vi "Acquire.vi"(8 "error in (no error)":errorcluster, 10 "Msg in":T1, 11 "PXIDigitizer in":refnum<class "PXIDigitizer.lvclass">) -> (0 "error out":errorcluster, 1 "new command":string, 2 "Msg out":T1, 3 "PXIDigitizer out":refnum<class "PXIDigitizer.lvclass">)   [LabVIEW 2011, in "PXIDigitizer.lvclass"]
uses:
  PXIDigitizer.lvclass
  DriverMsg.ctl
  PXIDigitizer.lvclass/PXIDigitizer.ctl
  BaseDriver/BaseDriver.lvclass
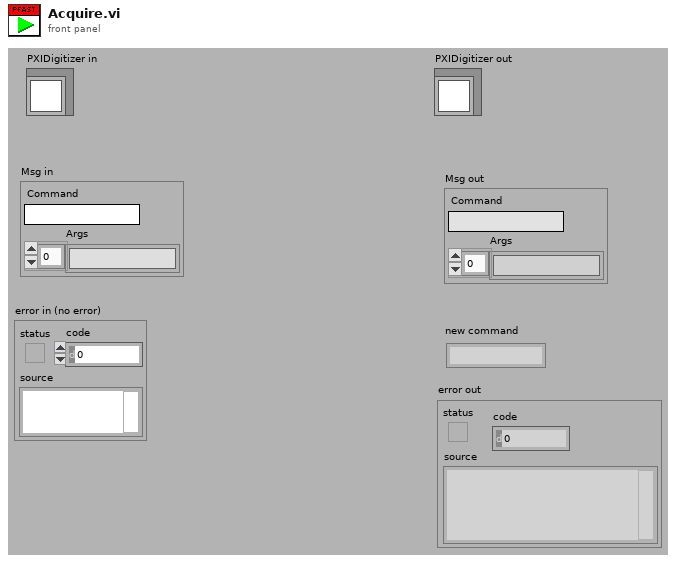
[diagram p1: front panel]
types:
  T1 = typedef "DriverMsg.ctl" = cluster{"Command":string, "Args":string[]}
  T2 = typedef "OnOffTypeDef.ctl" = enum16{"off", "on"}
  T3 = typedef "methodCluster_TypDEf.ctl" = cluster{"Analysis1":T4, "Analysis2":T4, "Analysis3":T4, "Analysis4":T4, "Analysis5":T4, "Analysis6":T4, "Analysis7":T4, "Analysis8":T4, "Analysis9":T4, "Analysis10":T4}
  T4 = typedef "method_TypDef.ctl" = enum16{"n/a", "max", "min", "energy"}
  T5 = typedef "LinkedChannelsCluster_TypDef.ctl" = cluster{"Analysis1":T6, "Analysis2":T6, "Analysis3":T6, "Analysis4":T6, "Analysis5":T6, "Analysis6":T6, "Analysis7":T6, "Analysis8":T6, "Analysis9":T6, "Analysis10":T6}
  T6 = typedef "channels_TypDef.ctl" = enum16{"Channel0", "Channel1", "Channel2", "Channel3", "Channel4", "Channel5", "Channel6", "Channel7", "n/a"}
  T7 = typedef "MeasurementsCluster_TypDEf.ctl" = cluster{"Analysis1":dbl, "Analysis2":dbl, "Analysis3":dbl, "Analysis4":dbl, "Analysis5":dbl, "Analysis6":dbl, "Analysis7":dbl, "Analysis8":dbl, "Analysis9":dbl, "Analysis10":dbl}
  T8 = cluster{"actualSamples":i32, "absoluteInitialX":dbl, "relativeInitialX":dbl, "xIncrement":dbl, "offset":dbl, "gain":dbl, "reserved1":dbl, "reserved2":dbl}[]
  T9 = cluster{"Channel0":string, "Channel1":string, "Channel2":string, "Channel3":string, "Channel4":string, "Channel5":string, "Channel6":string, "Channel7":string}
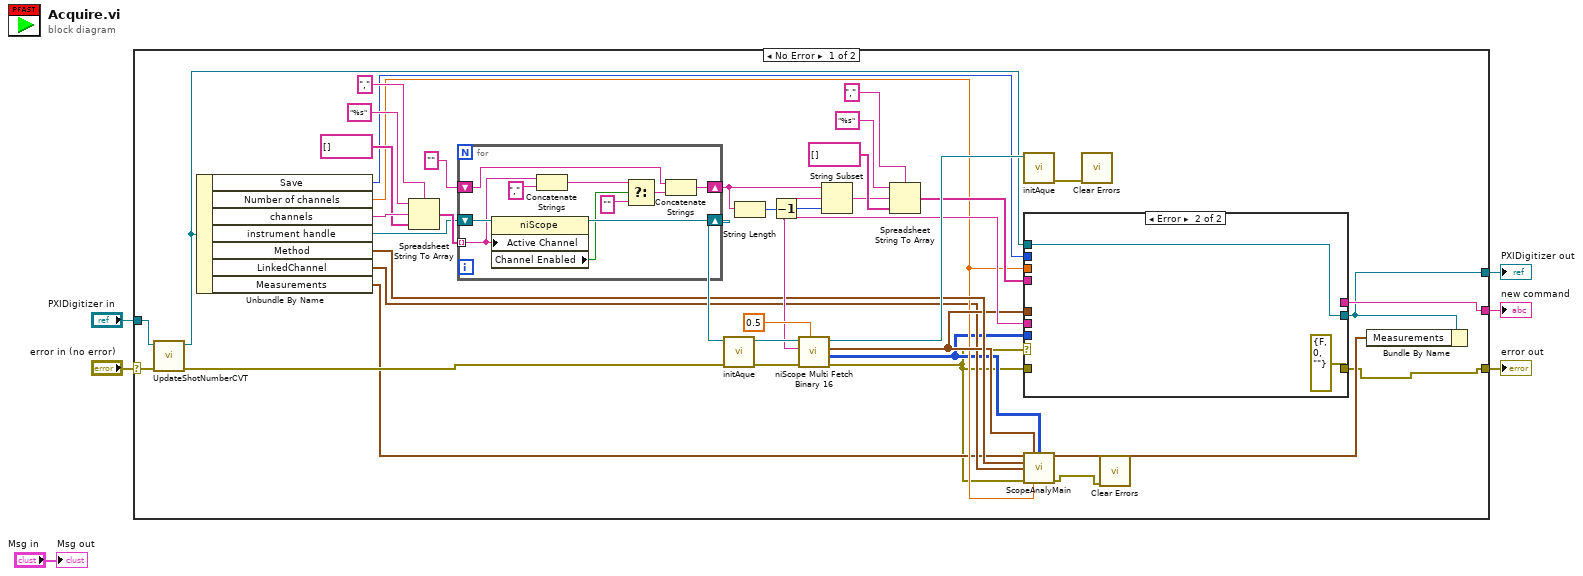
[diagram p0: block diagram]
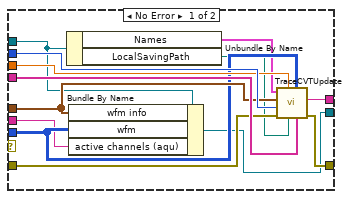
[diagram p2: hidden frame]
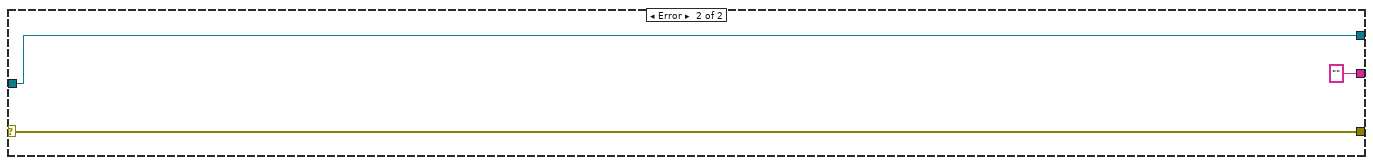
[diagram p3: hidden frame]
diagram:
  n1 = case shown="No Error" "error in (no error)" {
    selector: "error in (no error)" -> [w35 w71]
    tunnel: "PXIDigitizer in" -> [w44 w72]
    tunnel: [w11 w72] -> w6
    tunnel: [w7 w71] -> w4
    tunnel: [w22 "" ("new command")] -> w1
    frame No Error {
      n2 = call "UpdateShotNumberCVT.vi"("error in (no error)"=w35, "BaseDriver in"=w44) -> ("error out"=w43:errorcluster, "BaseDriver out"=w20:refnum<class "PXIDigitizer.lvclass">)  [unwired: 8 in]
      n3 = Unbundle By Name ("pressure read")(w20) -> ("Save"=w19:T2, "Number of channels"=w15:dbl, "channels"=w41:string, "instrument handle"=w18:refnum<k15>, "Method"=w17:T3, "LinkedChannel"=w14:T5, "Measurements"=w13:T7)
      n4 = Spreadsheet String To Array(delimiter (Tab)=",", format string="%s", spreadsheet string=w41, array type (2D Dbl)=string[] []) -> (array=w28:string[])
      n5 = for {
        shift-right: [w68] -> w24
        shift-left: w18 -> [w69]
        tunnel: w28 -> [w64] mode=indexing
        shift-right: [w61] -> w23
        shift-left: "" -> [w60]
        n6 = property class="niScope"(reference=w69, "Active Channel"=w64) -> (reference out=w68:refnum<k15>, "Channel Enabled"=w67:bool)  [unwired: 1 in, 1 out]
        n7 = Concatenate Strings(w64, "," ("string")) -> (w63:string)
        n8 = Select(t=w63, s=w67, f="") -> (s? t:f=w62:string)
        n9 = Concatenate Strings(w60, w62) -> (w61:string)
      }
      n10 = call "initAque.vi"("error in (no error)"=w43, "IVI Refnum in"=w24) -> ("error out"=w37:errorcluster, "IVI Refnum out"=w38:refnum<k15>)  [unwired: 8 in]
      n11 = String Length(string=w23) -> (length=w26:i32)
      n12 = Decrement(x=w26) -> (x-1=w25:i32)
      n13 = String Subset(string=w23, length (rest)=w25) -> (substring=w21:string)  [unwired: 1 in]
      n14 = call "niScope Multi Fetch Binary 16.vi"("timeout"=0.5, "error in"=w37, "channels"=w21, "instrument handle"=w38) -> ("error out"=w9:errorcluster, "wfm"=w12:i16[][], "wfm info"=w16:T8, "instrument handle out"=w36:refnum<k15>)  [unwired: 4 in]
      n15 = Spreadsheet String To Array(delimiter (Tab)=",", format string="%s", spreadsheet string=w21, array type (2D Dbl)=string[] []) -> (array=w33:string[])
      n16 = call "initAque.vi"("IVI Refnum in"=w36) -> ("error out"=w32:errorcluster)  [unwired: 9 in, 1 out]
      n17 = case shown="Error" w9 {
        tunnel: w33 -> [w57 _]
        tunnel: w9 -> [w56 _]
        tunnel: [w55 _] -> w22
        tunnel: [w54 errorcluster {"status"=FALSE, "code"=0, "source"=""} ("error out")] -> w7
        tunnel: [w48 w59] -> w11
        tunnel: w21 -> [w49 _]
        tunnel: w20 -> [w47 w59]
        tunnel: w19 -> [w53 _]
        tunnel: w12 -> [w50 _]
        tunnel: w16 -> [w51 _]
        tunnel: w15 -> [w52 _]
        frame No Error {
          n18 = Unbundle By Name ("pressure read")(w47) -> ("Names"=w46:T9, "LocalSavingPath"=w45:path)
          n19 = Bundle By Name(cluster=w47, "wfm info"=w51, "wfm"=w50, "active channels (aqu)"=w49) -> (w48:refnum<class "PXIDigitizer.lvclass">)
          n20 = call "TraceCVTUpdate.vi"("Array"=w57, "wfm"=w50, "Settings.LocalSavingPath"=w45, "Number of channels"=w52, "error in (no error)"=w56, "Save"=w53, "wfm info"=w51, "Settings.Names"=w46) -> ("error out"=w54:errorcluster, "String out"=w55:string)  [unwired: 1 in, 1 out]
        }
        frame Error {
        }
      }
      n21 = call "ScopeAnalyMain.vi"("Measurements"=w13, "wfm info"=w16, "wfm"=w12, "Method"=w17, "LinkedChannel"=w14, "error in (no error)"=w9, "Number of channels"=w15) -> ("Measurements"=w10:T7, "error out"=w8:errorcluster)  [unwired: 7 in]
      n22 = call "Clear Errors.vi"("error in (no error)"=w32) -> ()  [unwired: 6 in, 1 out]
      n23 = call "Clear Errors.vi"("error in (no error)"=w8) -> ()  [unwired: 6 in, 1 out]
      n24 = Bundle By Name(cluster=w11, "Measurements"=w10) -> ()  [unwired: 1 out]
    }
    frame Error {
    }
  }
  "PXIDigitizer out" <- w6
  "error out" <- w4
  "new command" <- w1
  "Msg out" <- "Msg in"
